vi "When Method One Return Value.vi"(2 "Return Value":dbl, 8 "error in (no error)":errorcluster, 11 "Test Interface Mock in":refnum<class "Test Interface Mock.lvclass">) -> (0 "error out":errorcluster, 3 "Test Interface Mock out":refnum<class "Test Interface Mock.lvclass">)   [LabVIEW 2020, in "Test Interface Mock.lvclass"]
uses:
  Test Interface Mock.lvclass
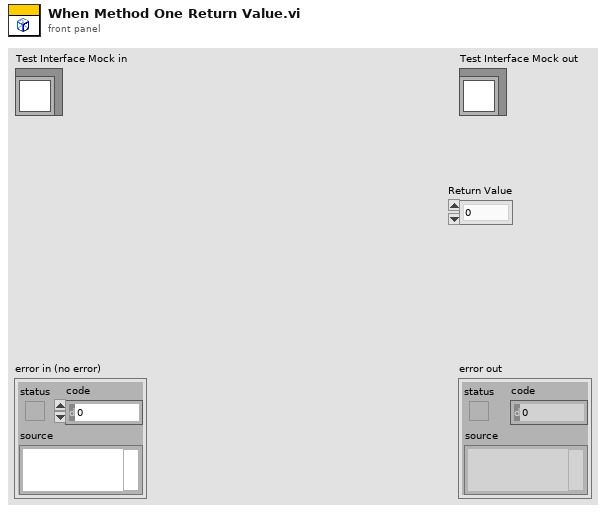
[diagram p1: front panel]
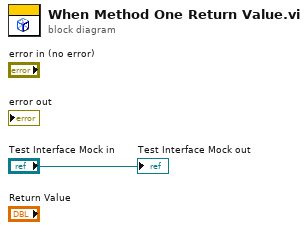
[diagram p0: block diagram]
diagram:
  "Test Interface Mock out" <- "Test Interface Mock in"
